vi "Caraya Test Example.vi"() -> ()   [LabVIEW 2013]
uses:
  <vilib>/LabVIEW Open Source Project/Cron Scheduler/Job/Job Report -- cluster.ctl
  Caraya Job Configuration -- cluster.ctl
  <vilib>/LabVIEW Open Source Project/Cron Scheduler/Job/Job.lvclass/Job.ctl
  <vilib>/LabVIEW Open Source Project/Cron Scheduler/JobReport/JobReport.lvclass/JobReport.ctl
  <vilib>/LabVIEW Open Source Project/Cron Scheduler/Cron/Create Cron Job.vi
  <vilib>/LabVIEW Open Source Project/Cron Scheduler/Cron/Compute Next Cron.vi
  <vilib>/LabVIEW Open Source Project/Cron Scheduler/Cron.Quartz/Cron.Quartz.lvclass
  <vilib>/LabVIEW Open Source Project/Cron Scheduler/Job/Job.lvclass
  <vilib>/LabVIEW Open Source Project/Cron Scheduler/openCron.lvlib
  <vilib>/LabVIEW Open Source Project/Cron Scheduler/JobReport/JobReport.lvclass
  <vilib>/LabVIEW Open Source Project/Cron Scheduler/Job.StaticVIRef/Job.StaticVIRef.lvclass
  <vilib>/addons/_JKI.lib/Serialization/JSON/JKI JSON Serialization.lvlib
panel:
  in  "Verbose (T)":bool=TRUE
  in  "Inspect Recursively (T)":bool=TRUE
  out "Report Path":path
  out "Test Path":path
  out "last error":errorcluster
  in  "Kill Job":bool
  in  "Abort Job":bool
  out "Job Report":T1
  out "Map":variant
  in  "Cron Expression":string="0/10 * * ? * *"
  out "syntax valid?":bool
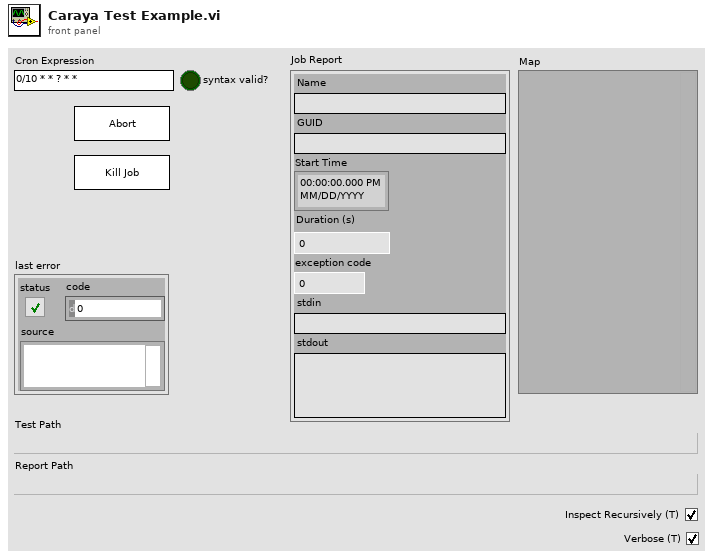
[diagram p1: front panel]
types:
  T1 = typedef "openCronJob.lvlib/JobReport.lvclass/Job Report -- cluster.ctl" = cluster{"Name":string, "GUID":string, "Start Time":timestamp, "Duration (s)":dbl, "exception code":i32, "stdin":string, "stdout":string}
  T2 = typedef "Caraya Job Configuration -- cluster.ctl" = cluster{"Test Path":path, "Report Path":path, "Inspect Recursively":bool, "Verbose":bool}
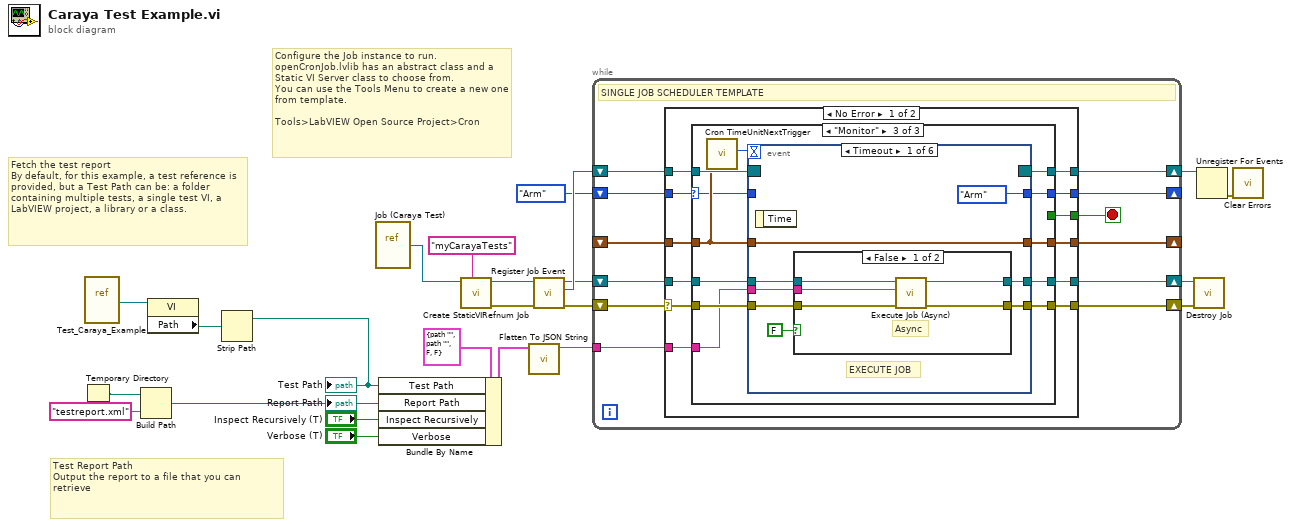
[diagram p0: block diagram]
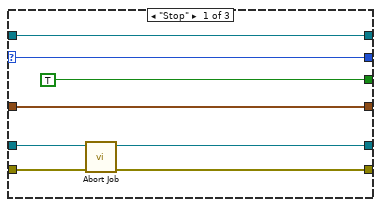
[diagram p2: hidden frame]
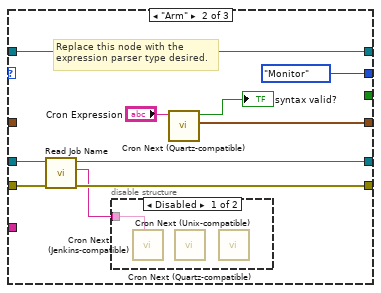
[diagram p3: hidden frame]
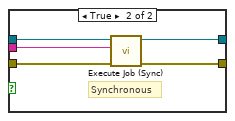
[diagram p5: hidden frame]
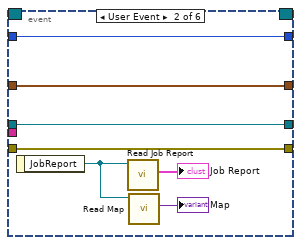
[diagram p6: hidden frame]
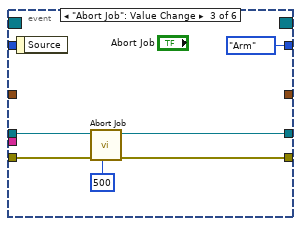
[diagram p7: hidden frame]
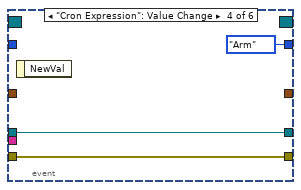
[diagram p8: hidden frame]
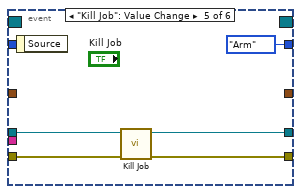
[diagram p9: hidden frame]
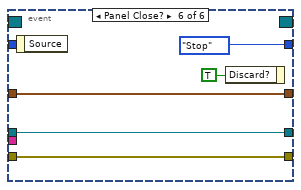
[diagram p10: hidden frame]
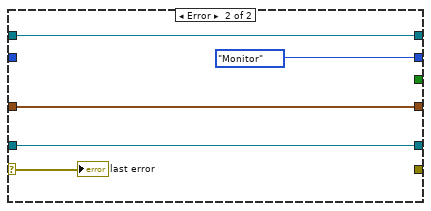
[diagram p11: hidden frame]
diagram:
  # "Test Report Path \nOutput the report to a file that you can retrieve"
  # "Fetch the test report \nBy default, for this example, a test reference is provided, but a Test Path can be: a folder containing multiple tests, a single test VI, a LabVIEW project, a library or a class."
  # "Configure the Job instance to run.\nopenCronJob.lvlib has an abstract class and a Static VI Server class to choose from.\nYou can use the Tools Menu to create a new one from template.\n\nTools>LabVIEW Open Source Project>Cron"
  n1 = Temporary Directory() -> (w3:path)
  n2 = vi-ref "Test_Caraya_Example.vi"() -> (w6:refnum<vi>)
  n3 = Build Path(base path=w3, name or relative path="testreport.xml") -> (appended path=w2:path)
  "Report Path" <- w2
  n4 = property class="VI"(reference=w6) -> ("Path"=w5:path)  [unwired: 1 in, 2 out]
  n5 = Strip Path(path=w5) -> (stripped path=w4:path)  [unwired: 1 out]
  "Test Path" <- w4
  n6 = vi-ref "Job (Caraya Test).vi"() -> (w22:refnum<vi>)
  n7 = Bundle By Name(cluster=T2 {"Test Path"=path "", "Report Path"=path "", "Inspect Recursively"=FALSE, "Verbose"=FALSE} ("Test Config"), "Test Path"=w4, "Report Path"=w2, "Inspect Recursively"="Inspect Recursively (T)", "Verbose"="Verbose (T)") -> (w10:T2)
  n8 = call <vilib>:"Create StaticVIRefnum Job.vi"("Job Name"="myCarayaTests", "Static VI Refnum"=w22) -> ("error out"=w18:errorcluster, "Job.StaticVIRef out"=w16:refnum<class "Job.StaticVIRef.lvclass">)  [unwired: 8 in]
  n9 = call <vilib>:"Flatten To JSON String.vi"("Variant"=w10) -> ("JSON String"=w9:string)  [unwired: 9 in, 1 out]
  n10 = call <vilib>:"Register Job Event.vi"("Job in"=w16) -> ("Job Event Registration"=w20:refnum<event-registration>, "Job out"=w17:refnum<class "Job.StaticVIRef.lvclass">)  [unwired: 9 in]
  n11 = while {
    shift-right: [w33] -> _
    shift-left: _ -> [w34]
    shift-right: [w31] -> _
    shift-left: enum16{"Arm", "Stop", "Monitor"}."Arm" -> [w32]
    shift-right: [w28] -> w13
    shift-left: w20 -> [w29]
    shift-right: [w26] -> w15
    shift-left: w17 -> [w27]
    shift-right: [w25] -> w19
    shift-left: w18 -> [w24]
    tunnel: w9 -> [w23]
    stop <- w30 stop-if-true
    # "SINGLE JOB SCHEDULER TEMPLATE"
    n12 = case shown="No Error" w24 {
      selector: w24 -> [w36 w122]
      tunnel: w34 -> [w46 w124]
      tunnel: [w45 w124] -> w33
      tunnel: w32 -> [w44 _]
      tunnel: [w43 enum16{"Arm", "Stop", "Monitor"}."Monitor"] -> w31
      tunnel: [w42 _] -> w30
      tunnel: w29 -> [w41 w126]
      tunnel: [w40 w126] -> w28
      tunnel: w27 -> [w39 w123]
      tunnel: [w38 w123] -> w26
      tunnel: [w37 _] -> w25
      tunnel: w23 -> [w35 _]
      frame No Error {
        n13 = case shown="\"Monitor\"" w44 {
          selector: w44 -> [w54 _ w69]
          tunnel: w46 -> [w52 _ w72]
          tunnel: [w52 w63 w74] -> w45
          tunnel: [w54 enum16{"Arm", "Stop", "Monitor"}."Monitor" w75] -> w43
          tunnel: [TRUE _ _] -> w42
          tunnel: w41 -> [w51 w64 w77]
          tunnel: [w51 w64 w76] -> w40
          tunnel: w39 -> [w50 w57 w71]
          tunnel: [w49 w56 w70] -> w38
          tunnel: w36 -> [w48 w59 w68]
          tunnel: [w47 w58 w67] -> w37
          tunnel: w35 -> [_ _ w66]
          frame "Stop" {
            n14 = call <vilib>:"Abort Job.vi"("error in (no error)"=w48, "Job in"=w50) -> ("error out"=w47:errorcluster, "Job out"=w49:refnum<class "Job.StaticVIRef.lvclass">)  [unwired: 5 in, 3 out]
          }
          frame "Arm" {
            # "Replace this node with the\nexpression parser type desired."
            n15 = call <vilib>:"Read Job Name.vi"("error in (no error)"=w59, "Job in"=w57) -> ("error out"=w58:errorcluster, "Name"=w55:string, "Job out"=w56:refnum<class "Job.StaticVIRef.lvclass">)  [unwired: 7 in]
            n16 = disable-structure shown="Disabled" {
              disable-tunnel: w55 -> [w65 _]
              frame Disabled {
                n17 = call <vilib>:"Cron Next (Jenkins-compatible).vi"("Job Name"=w65) -> ()  [unwired: 8 in, 3 out]
                n18 = call <vilib>:"Cron Next (Quartz-compatible).vi"() -> ()  [unwired: 9 in, 3 out]
                n19 = call <vilib>:"Cron Next (Unix-compatible).vi"() -> ()  [unwired: 9 in, 3 out]
              }
              frame Enabled {
              }
            }
            n20 = call <vilib>:"Cron Next (Quartz-compatible).vi"("Cron Expression"="Cron Expression") -> ("Next Occurence"=w63:timestamp, "syntax valid?"=→"syntax valid?":bool)  [unwired: 8 in, 1 out]
          }
          frame "Monitor" {
            n21 = call <vilib>:"Cron TimeUnitNextTrigger.vi"("Next Occurence"=w72) -> ("next event (ms)"=w73:i32)  [unwired: 10 in]
            n22 = event shown="[0] Timeout" {
              selector: w77 -> [_ _ _ _ _ _]
              dyn-events: [_ _ _ _ _ _] -> w76
              timeout: w73 -> [_ _ _ _ _ _]
              tunnel: [enum16{"Arm", "Stop", "Monitor"}."Arm" w101 enum16{"Arm", "Stop", "Monitor"}."Arm" enum16{"Arm", "Stop", "Monitor"}."Arm" enum16{"Arm", "Stop", "Monitor"}."Arm" enum16{"Arm", "Stop", "Monitor"}."Stop"] -> w75
              tunnel: [w79 w102 _ _ _ w119] -> w74
              tunnel: w72 -> [w79 w102 _ _ _ w119]
              tunnel: w71 -> [w84 w100 w107 w110 w115 w118]
              tunnel: [w82 w100 w106 w110 w114 w118] -> w70
              tunnel: w69 -> [_ w101 _ _ _ _]
              tunnel: w68 -> [w81 w99 w104 w109 w113 w117]
              tunnel: [w80 w99 w103 w109 w112 w117] -> w67
              tunnel: w66 -> [w78 _ _ _ _ _]
              event Timeout {
                # "EXECUTE JOB"
                n23 = event-data() -> ()  [unwired: 1 in, 1 out]
                n24 = case shown="False" FALSE ("Synchronous?") {
                  tunnel: w84 -> [w90 w95]
                  tunnel: [w89 w94] -> w82
                  tunnel: w81 -> [w87 w93]
                  tunnel: [w88 w92] -> w80
                  tunnel: w78 -> [w86 w91]
                  frame False {
                    # "Async"
                    n25 = call <vilib>:"Execute Job (Async).vi"("error in (no error)"=w87, "stdin"=w86, "Job in"=w90) -> ("error out"=w88:errorcluster, "Job out"=w89:refnum<class "Job.StaticVIRef.lvclass">)  [unwired: 6 in, 1 out]
                  }
                  frame True {
                    # "Synchronous"
                    n26 = call <vilib>:"Execute Job (Sync).vi"("error in (no error)"=w93, "stdin"=w91, "Job in"=w95) -> ("error out"=w92:errorcluster, "Job out"=w94:refnum<class "Job.StaticVIRef.lvclass">)  [unwired: 5 in, 2 out]
                  }
                }
              }
              event User Event {
                n27 = event-data() -> ("JobReport"=w97:refnum<class "JobReport.lvclass">)  [unwired: 1 in]
                n28 = call <vilib>:"Read Job Report.vi"("JobReport in"=w97) -> ("Job Report"=→"Job Report":T1)  [unwired: 8 in, 2 out]
                n29 = call <vilib>:"Read Map.vi"("JobReport in"=w97) -> ("Map"=→"Map":variant)  [unwired: 8 in, 2 out]
              }
              event "Abort Job": Value Change {
                n30 = event-data() -> ()  [unwired: 1 in, 1 out]
                n31 = call <vilib>:"Abort Job.vi"("timeout (500 ms)"=500, "error in (no error)"=w104, "Job in"=w107) -> ("error out"=w103:errorcluster, "Job out"=w106:refnum<class "Job.StaticVIRef.lvclass">)  [unwired: 4 in, 3 out]
              }
              event "Cron Expression": Value Change {
                n32 = event-data() -> ()  [unwired: 1 in, 1 out]
              }
              event "Kill Job": Value Change {
                n33 = event-data() -> ()  [unwired: 1 in, 1 out]
                n34 = call <vilib>:"Kill Job.vi"("error in (no error)"=w113, "Job in"=w115) -> ("error out"=w112:errorcluster, "Job out"=w114:refnum<class "Job.StaticVIRef.lvclass">)  [unwired: 8 in]
              }
              event Panel Close? {
                n35 = event-data() -> ()  [unwired: 1 in, 1 out]
                n36 = event-data("Discard?"=TRUE) -> ()  [unwired: 1 in, 1 out]
              }
            }
          }
        }
      }
      frame Error {
        "last error" <- w122
      }
    }
  }
  n37 = call <vilib>:"Destroy Job.vi"("error in (no error)"=w19, "Job in"=w15) -> ()  [unwired: 8 in, 2 out]
  n38 = Unregister For Events(event registration refnum=w13) -> (error out=w14:errorcluster)  [unwired: 1 in]
  n39 = call <vilib>:"Clear Errors.vi"("error in (no error)"=w14) -> ()  [unwired: 6 in, 1 out]
